vi "Read-Only Stats.vi"() -> (0 "Collisions":i32[](array[numeric]), 1 "Kills":i32[](array[numeric]), 2 "Generated":i32[](array[numeric]), 3 "Squares":i32[](array[numeric]))   [LabVIEW 2015, in "SB SubVIs.lvlib"]
uses:
  SB SubVIs.lvlib
  Globals (private).vi
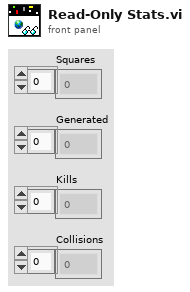
[diagram p1: front panel]
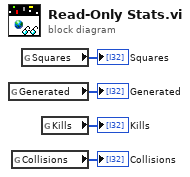
[diagram p0: block diagram]
diagram:
  n1 = global read "Globals (private).vi" "Generated"() -> (→"Generated":i32[])
  n2 = global read "Globals (private).vi" "Collisions"() -> (→"Collisions":i32[])
  n3 = global read "Globals (private).vi" "Squares"() -> (→"Squares":i32[])
  n4 = global read "Globals (private).vi" "Kills"() -> (→"Kills":i32[])
